vi "ChatCypher.vi"() -> ()   [LabVIEW 2022 SP3]
panel:
  out "Coded":string
  in  "Original":string
  out "Decoded":string
  in  "Cyphered":string
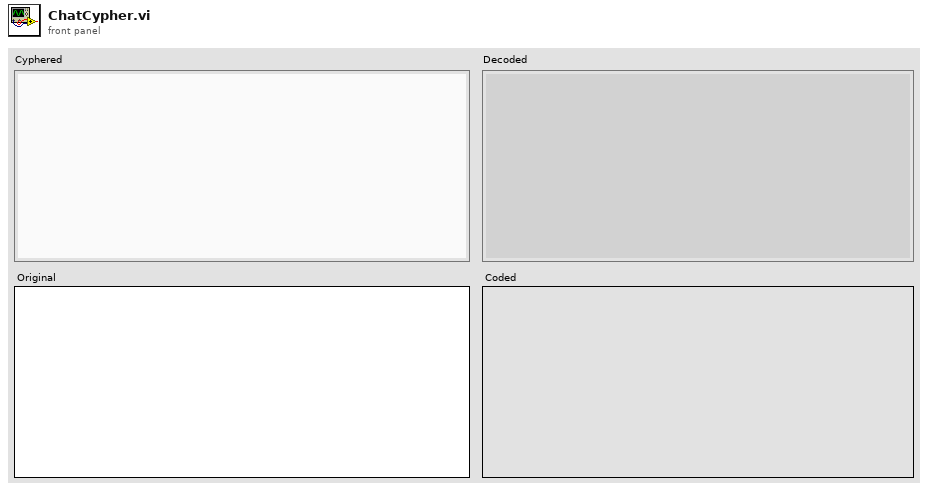
[diagram p1: front panel]
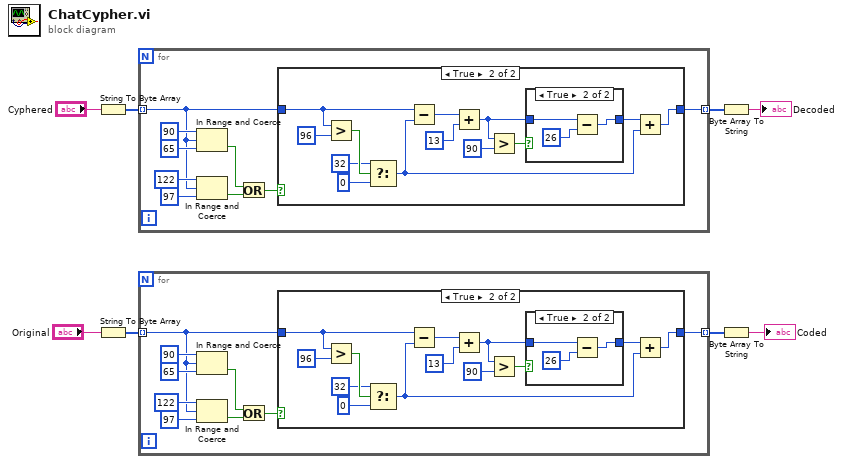
[diagram p0: block diagram]
diagram:
  n1 = String To Byte Array(string="Cyphered") -> (unsigned byte array=w7:u8[])
  n2 = String To Byte Array(string="Original") -> (unsigned byte array=w3:u8[])
  n3 = for {
    tunnel: w7 -> [w12] mode=indexing
    tunnel: [w17] -> w6 mode=indexing
    n4 = In Range and Coerce(upper limit=u8 90, x=w12, lower limit=u8 65) -> (In Range?=w10:bool)  [unwired: 1 out]
    n5 = In Range and Coerce(upper limit=u8 122, x=w12, lower limit=u8 97) -> (In Range?=w11:bool)  [unwired: 1 out]
    n6 = Or(x=w10, y=w11) -> (x .or. y?=w9:bool)
    n7 = case shown="True" w9 {
      tunnel: [w18 w20] -> w17
      tunnel: w12 -> [w18 w19]
      frame False {
      }
      frame True {
        n8 = Greater?(x=w19, y=u8 96) -> (0:w30:bool)
        n9 = Select(t=u8 32 ("y"), s=w30, f=u8 0) -> (s? t:f=w21:u8)
        n10 = Subtract(x=w19, y=w21) -> (x-y=w26:u8)
        n11 = Add(x=w26, y=u8 13) -> (x+y=w23:u8)
        n12 = Greater?(x=w23, y=u8 90) -> (0:w24:bool)
        n13 = case shown="True" w24 {
          tunnel: w23 -> [w32 w35]
          tunnel: [w32 w33] -> w22
          frame False {
          }
          frame True {
            n14 = Subtract(x=w35, y=u8 26) -> (x-y=w33:u8)
          }
        }
        n15 = Add(x=w22, y=w21) -> (x+y=w20:u8)
      }
    }
  }
  n16 = for {
    tunnel: w3 -> [w39] mode=indexing
    tunnel: [w44] -> w4 mode=indexing
    n17 = In Range and Coerce(upper limit=u8 90, x=w39, lower limit=u8 65) -> (In Range?=w37:bool)  [unwired: 1 out]
    n18 = In Range and Coerce(upper limit=u8 122, x=w39, lower limit=u8 97) -> (In Range?=w38:bool)  [unwired: 1 out]
    n19 = Or(x=w37, y=w38) -> (x .or. y?=w36:bool)
    n20 = case shown="True" w36 {
      tunnel: [w45 w47] -> w44
      tunnel: w39 -> [w45 w46]
      frame False {
      }
      frame True {
        n21 = Greater?(x=w46, y=u8 96) -> (0:w57:bool)
        n22 = Select(t=u8 32 ("y"), s=w57, f=u8 0) -> (s? t:f=w48:u8)
        n23 = Subtract(x=w46, y=w48) -> (x-y=w53:u8)
        n24 = Add(x=w53, y=u8 13) -> (x+y=w50:u8)
        n25 = Greater?(x=w50, y=u8 90) -> (0:w51:bool)
        n26 = case shown="True" w51 {
          tunnel: w50 -> [w59 w62]
          tunnel: [w59 w60] -> w49
          frame False {
          }
          frame True {
            n27 = Subtract(x=w62, y=u8 26) -> (x-y=w60:u8)
          }
        }
        n28 = Add(x=w49, y=w48) -> (x+y=w47:u8)
      }
    }
  }
  n29 = Byte Array To String(unsigned byte array=w6) -> (string=→"Decoded":string)
  n30 = Byte Array To String(unsigned byte array=w4) -> (string=→"Coded":string)
